vi "PCinfo_XP.vi"(10 "DLL基路径":path) -> (2 "PC验证结果":bool)   [LabVIEW 2010]
panel:
  in  "PCinfoProject._CpuHdMac":refnum<k7> caption="PowerPoint._Application"
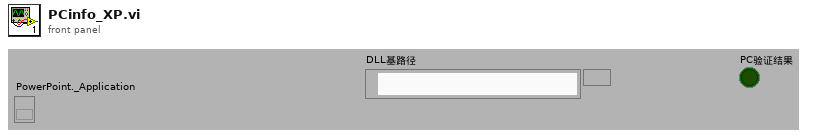
[diagram p1: front panel]
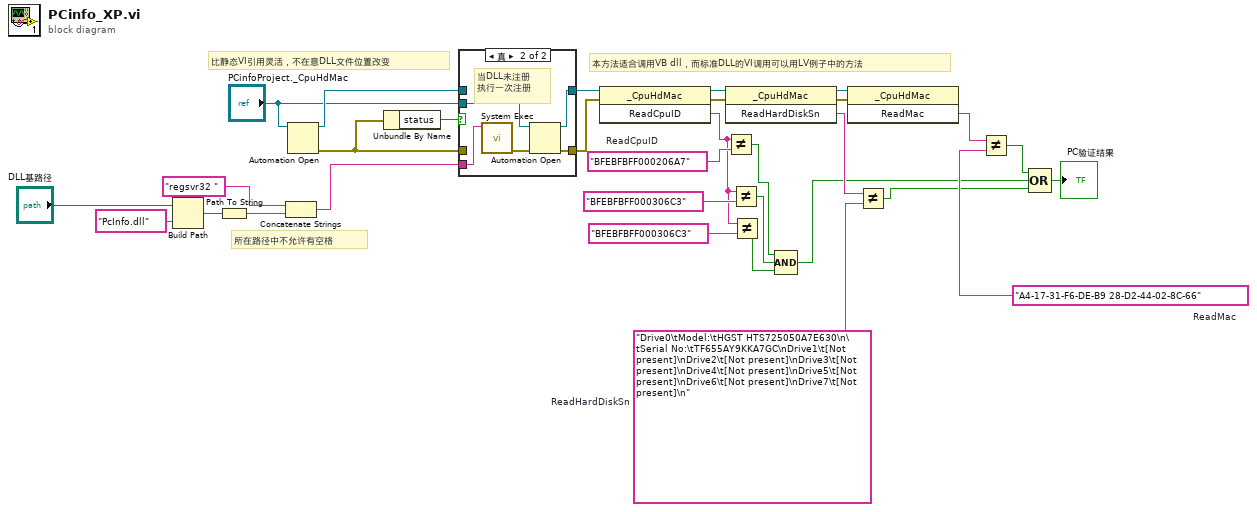
[diagram p0: block diagram]
diagram:
  w13 = "A4-17-31-F6-DE-B9 28-D2-44-02-8C-66"  # ReadMac
  w15 = "Drive0\tModel:\tHGST HTS725050A7E630\n\tSerial No:\tTF655AY9KKA7GC\nDrive1\t[Not present]\nDrive2\t[Not present]\nDrive3\t[Not present]\nDrive4\t[Not present]\nDrive5\t[Not present]\nDrive6\t[Not present]\nDrive7\t[Not present]\n"  # ReadHardDiskSn
  w16 = "BFEBFBFF000206A7"  # ReadCpuID
  # "所在路径中不允许有空格"
  # "比静态VI引用灵活，不在意DLL文件位置改变"
  # "本方法适合调用VB dll，而标准DLL的VI调用可以用LV例子中的方法"
  n1 = Build Path(base path="DLL基路径", name or relative path="PcInfo.dll" ("command line")) -> (appended path=w21:path)
  n2 = Path To String(path=w21) -> (string=w19:string)
  n3 = Concatenate Strings("regsvr32 " ("字符串"), w19) -> (w18:string)
  n4 = Automation Open(Automation Refnum="PCinfoProject._CpuHdMac") -> (Automation Refnum=w30:refnum<k7>, error out=w31:errorcluster)  [unwired: 3 in]
  n5 = Unbundle By Name(w31) -> ("status"=w29:bool)
  n6 = case shown="真" w29 {
    tunnel: [w32 w36] -> w27
    tunnel: w31 -> [w32 _]
    tunnel: w30 -> [w33 _]
    tunnel: [w33 w35] -> w28
    tunnel: "PCinfoProject._CpuHdMac" -> [_ w37]
    tunnel: w18 -> [_ w34]
    frame False {
    }
    frame True {
      # "当DLL未注册\n执行一次注册"
      n7 = call <vilib>:"System Exec.vi"("command line"=w34) -> ("error out"=w38:errorcluster)  [unwired: 7 in, 3 out]
      n8 = Automation Open(error in (no error)=w38, Automation Refnum=w37) -> (Automation Refnum=w35:refnum<k7>, error out=w36:errorcluster)  [unwired: 2 in]
    }
  }
  n9 = invoke class="_CpuHdMac" method="ReadCpuID"(reference=w28, error in=w27) -> (reference out=w26:refnum<k7>, error out=w25:errorcluster, "ReadCpuID"=w7:string)  [unwired: 1 in]
  n10 = invoke class="_CpuHdMac" method="ReadHardDiskSn"(reference=w26, error in=w25) -> (reference out=w24:refnum<k7>, error out=w23:errorcluster, "ReadHardDiskSn"=w14:string)  [unwired: 1 in]
  n11 = Not Equal?(x=w7, y=w16) -> (x != y?=w6:bool)
  n12 = Not Equal?(x=w7, y="BFEBFBFF000306C3" ("ReadCpuID")) -> (x != y?=w5:bool)
  n13 = Not Equal?(x=w7, y="BFEBFBFF000306C3" ("ReadCpuID")) -> (x != y?=w4:bool)
  n14 = Compound Arithmetic op=AND(w6, w5, w4) -> (w3:bool)
  n15 = invoke class="_CpuHdMac" method="ReadMac"(reference=w24, error in=w23) -> ("ReadMac"=w12:string)  [unwired: 1 in, 2 out]
  n16 = Not Equal?(x=w14, y=w15) -> (x != y?=w1:bool)
  n17 = Not Equal?(x=w12, y=w13) -> (x != y?=w2:bool)
  n18 = Compound Arithmetic op=OR(w2, w3, w1) -> (→"PC验证结果":bool)
